vi "数据存储-9205电压.vi"(8 "错误输入（无错误）":errorcluster, 10 "9205电压数据":waveform(dbl)[](array[waveform]), 11 "tdms文件输入":refnum<k34>) -> (0 "错误输出":errorcluster, 3 "tdms文件输出":refnum<k34>)   [LabVIEW 2013]
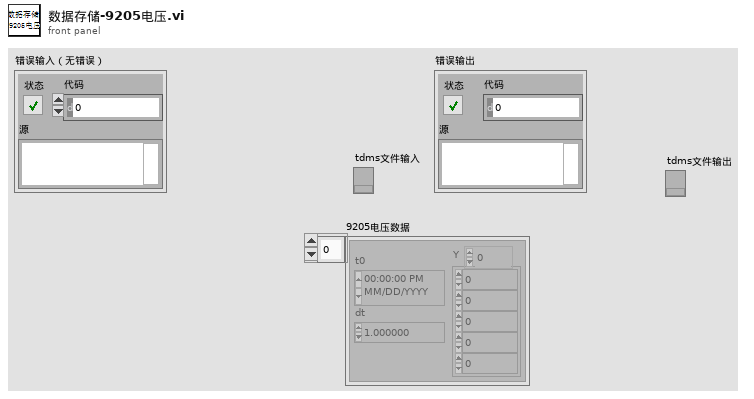
[diagram p1: front panel]
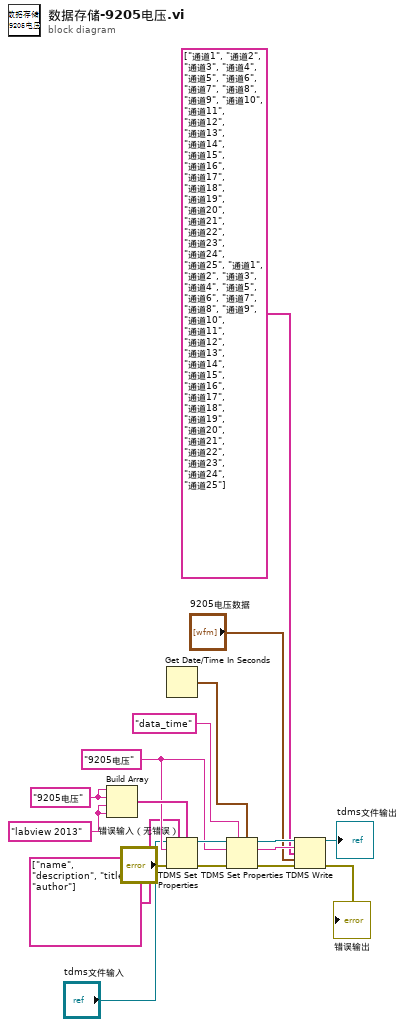
[diagram p0: block diagram]
diagram:
  w13 = "9205电压" ("组名称")
  w14 = "9205电压" ("9213")
  w18 = "labview 2013"
  n1 = Build Array(w14, w14, w18, w18) -> (w17:string[])
  n2 = Get Date/Time In Seconds() -> (seconds since 1Jan1904=w12:timestamp)
  n3 = TDMS Set Properties(5:w17, 7:string[] ["name", "description", "title", "author"] ("属性名称"), 8:"错误输入（无错误）", 10:w13, 11:"tdms文件输入") -> (0:w15:errorcluster, 3:w16:refnum<k34>)  [unwired: 1 in, 2 out]
  n4 = TDMS Set Properties(5:w12, 7:"data_time" ("属性名称"), 8:w15, 10:w13, 11:w16) -> (0:w8:errorcluster, 2:w9:string, 3:w10:refnum<k34>)  [unwired: 1 in, 1 out]
  n5 = TDMS Write(0:w10, 5:w9, 7:string[] ["通道1", "通道2", "通道3", "通道4", "通道5", "通道6", "通道7", "通道8", "通道9", "通道10", "通道11", "通道12", "通道13", "通道14", "通道15", "通道16", "通道17", "通道18", "通道19", "通道20", "通道21", "通道22", "通道23", "通道24", "通道25", "通道1", "通道2", "通道3", "通道4", "通道5", "通道6", "通道7", "通道8", "通道9", "通道10", "通道11", "通道12", "通道13", "通道14", "通道15", "通道16", "通道17", "通道18", "通道19", "通道20", "通道21", "通道22", "通道23", "通道24", "通道25"] ("通道名输入（无标题）"), 9:"9205电压数据", 11:w8) -> (4:→"tdms文件输出":refnum<k34>, 15:→"错误输出":errorcluster)  [unwired: 1 in, 2 out]
